vi "ari_mean.vi"() -> ()   [LabVIEW 2021]
panel:
  in  "Array":dbl[](array[numeric])
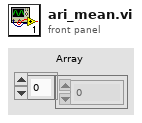
[diagram p1: front panel]
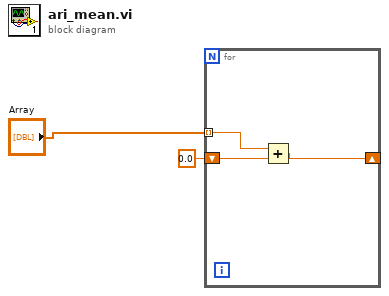
[diagram p0: block diagram]
diagram:
  n1 = for {
    tunnel: "Array" -> [w5] mode=indexing
    shift-right: [w4] -> _
    shift-left: 0.0 -> [w3]
    n2 = Add(x=w5, y=w3) -> (x+y=w4:dbl)
  }
